vi "IAmGLF-DeleteFromStandaloneProcess.vi"(8 "error in (no error)":errorcluster, 10 "Error Return Notifier":refnum<notifier>, 11 "IUseDVRHandler in":refnum<class "IUseDVRHandler.lvclass">) -> (0 "error out":errorcluster)   [LabVIEW 2024, in "GLF.lvlib" / "IUseDVRHandler.lvclass"]
uses:
  IUseDVRHandler.lvclass
  DVRHandler/DVRHandler.lvlib
  C:/Users/Thomas/Documents/Projects/GLF/Sources/GLF/IUseDVRHandler/IUseDVRHandler.lvclass
  C:/Users/Thomas/Documents/Projects/GLF/Sources/GLF/IAmGLF/IAmGLF.lvclass
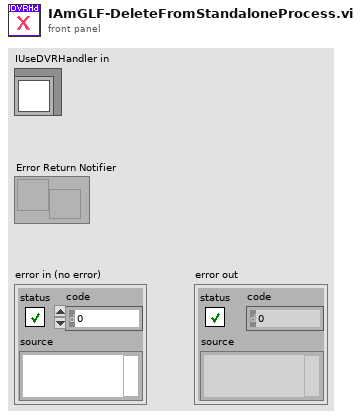
[diagram p1: front panel]
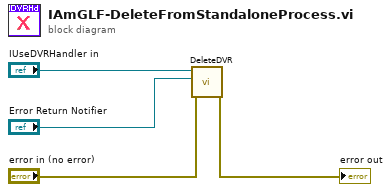
[diagram p0: block diagram]
diagram:
  n1 = call "DeleteDVR.vi"("error in (no error)"="error in (no error)", "Error Return Notifier"="Error Return Notifier", "IAmGLF To Create DVR"="IUseDVRHandler in") -> ("error out"=→"error out":errorcluster)  [unwired: 8 in]
